vi "AcquireSampleImages.vi"(6 "SampleName":string, 7 "TLCamera reference in":refnum<k24>, 8 "Error In":errorcluster, 9 "Exposure":u16, 10 "Schedule File":path, 11 "MotorController in":refnum<class "MotorController.lvclass">) -> (0 "Error Out":errorcluster, 3 "MotorController out":refnum<class "MotorController.lvclass">, 5 "TLCamera reference out":refnum<k24>)   [LabVIEW 2019]
uses:
  MotorController.lvclass
  C:/Users/jleeman/git_repos/CAxis_Machine/C-Axis LabView Controller/Library_X64/Thorlabs.TSI.TLCameraInterfaces.dll
  Library_X64/Thorlabs.TSI.TLCameraInterfaces.dll
  AcquireSampleImages_states_enum_typedef.ctl
  <vilib>/Utility/file.llb/Read Delimited Spreadsheet (I64).vi
panel:
  in  "Next":bool
  out "Progress":u8(slide) scale=0.0..100.0
  out "Image":u16[][](graph)
  out "Acquisition Schedule":i64[][](array[numeric])
  # "Measure Sample"
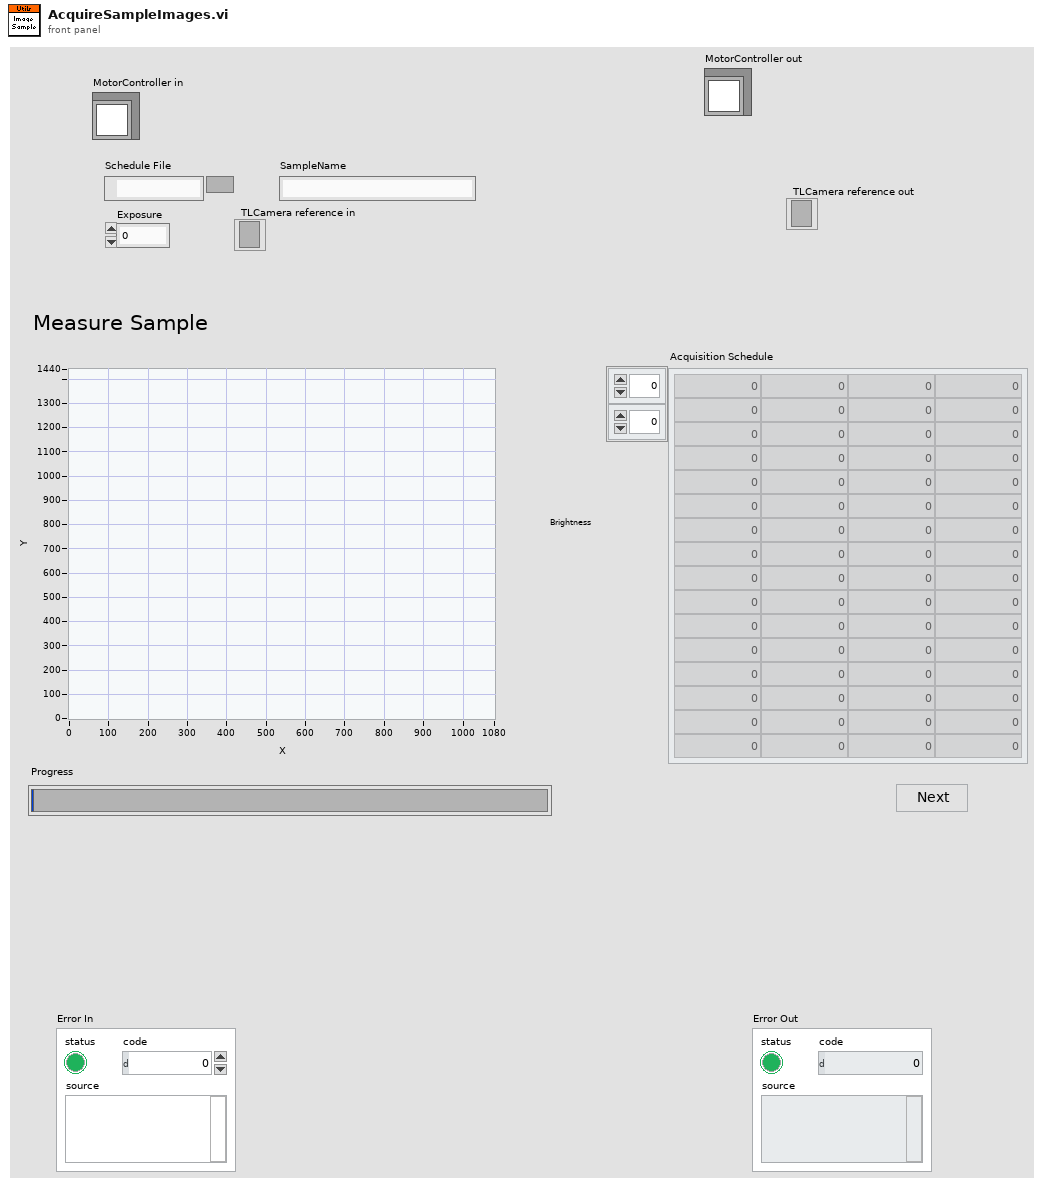
[diagram p1: front panel]
types:
  T1 = enum8{"Enabled", "Disabled", "Disabled and Grayed Out"}
  T2 = typedef "AcquireSampleImages_states_enum_typedef.ctl" = enum16{"Shutdown", "Wait", "TakeImages", "Initialize"}
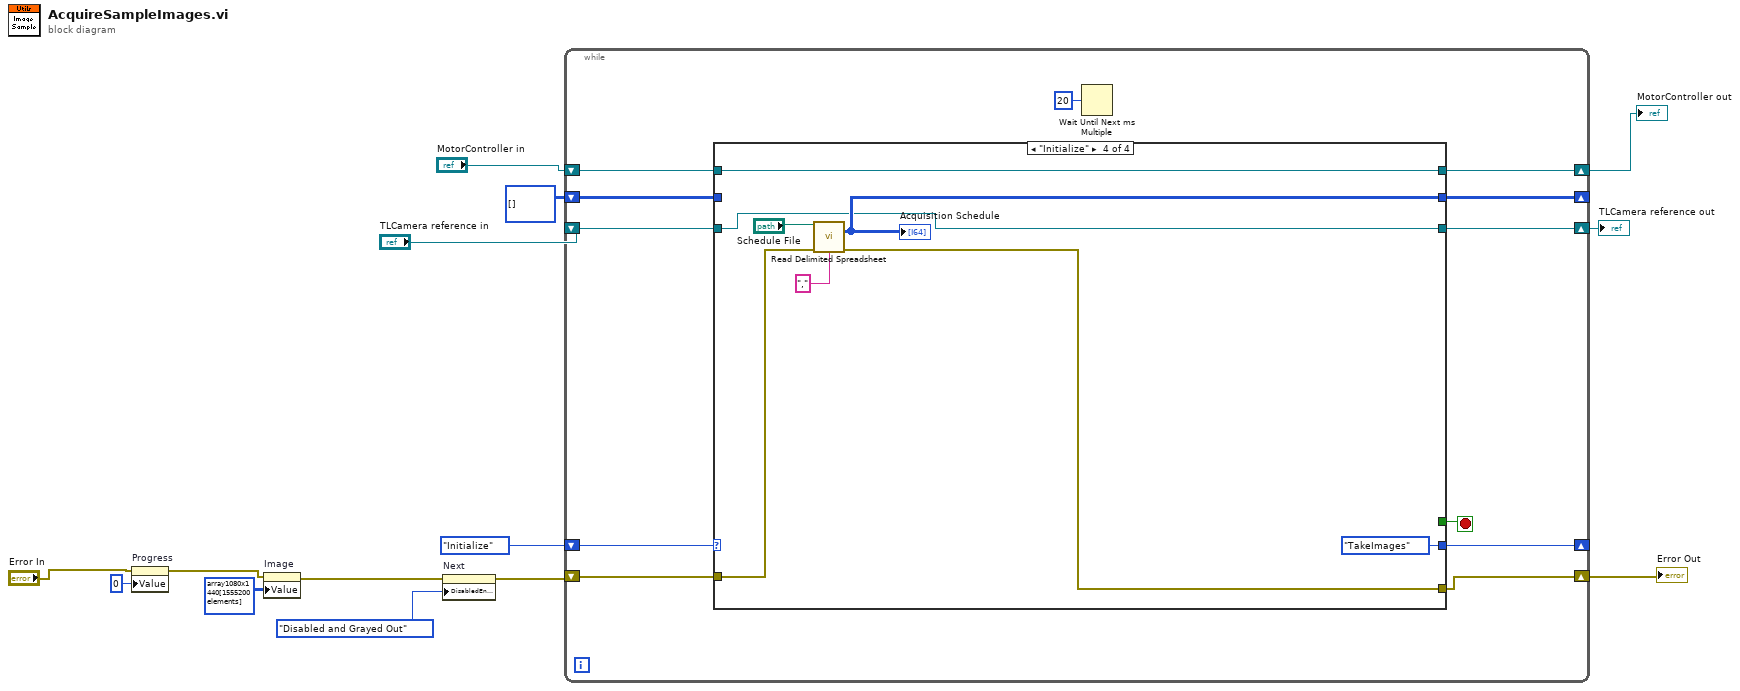
[diagram p0: block diagram]
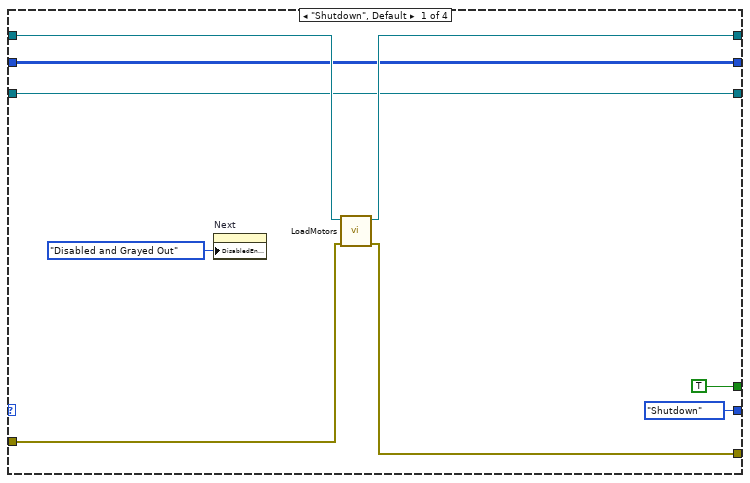
[diagram p2: hidden frame]
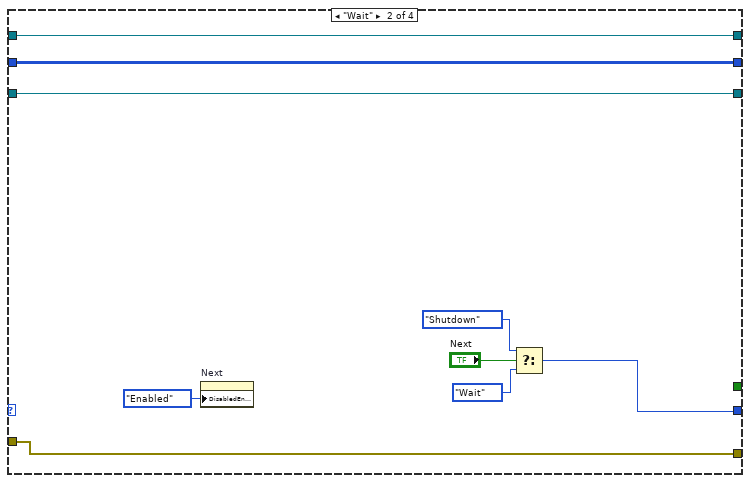
[diagram p3: hidden frame]
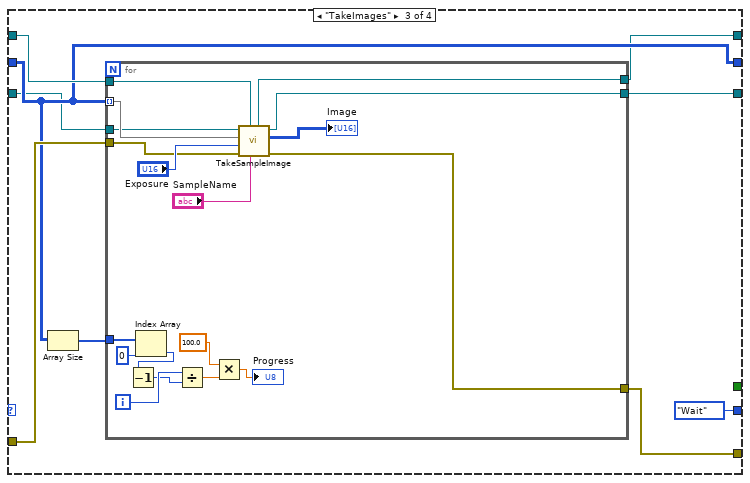
[diagram p4: hidden frame]
diagram:
  n1 = property on="Progress" class="Slide (strict)"(error in="Error In", "Value"=u8 0 ("Progress")) -> (error out=w5:errorcluster)  [unwired: 1 in, 1 out]
  n2 = property on="Image" class="IntGraph (strict)"(error in=w5, "Value"=u16[][] array1080x1440[1555200 elements] ("Image")) -> (error out=w4:errorcluster)  [unwired: 1 in, 1 out]
  n3 = property on="Next" class="Bool"(error in=w4, "DisabledEnum"=T1."Disabled and Grayed Out" ("Disabled")) -> (error out=w12:errorcluster)  [unwired: 1 in, 1 out]
  n4 = while {
    shift-right: [w25] -> _
    shift-left: AcquireSampleImages_states_enum_typedef."Initialize" -> [w26]
    shift-right: [w24] -> _
    shift-left: i64[][] [] ("all rows") -> [w21]
    shift-right: [w22] -> w8
    shift-left: w12 -> [w23]
    shift-right: [w20] -> w10
    shift-left: "MotorController in" -> [w19]
    shift-right: [w18] -> w1
    shift-left: "TLCamera reference in" -> [w17]
    stop <- w15 stop-if-true
    n5 = case shown="\"Initialize\"" w26 {
      tunnel: [AcquireSampleImages_states_enum_typedef."Shutdown" ("f") w41 AcquireSampleImages_states_enum_typedef."Wait" ("f") AcquireSampleImages_states_enum_typedef."TakeImages" ("f")] -> w25
      tunnel: [w31 w40 w49 w76] -> w24
      tunnel: w23 -> [w33 w36 w50 w77]
      tunnel: [w28 w36 w47 w73] -> w22
      tunnel: w21 -> [w31 w40 w49 _]
      tunnel: [w35 w38 w48 w75] -> w20
      tunnel: w19 -> [w34 w38 w51 w75]
      tunnel: [w29 w39 w45 w72] -> w18
      tunnel: w17 -> [w29 w39 w46 w72]
      tunnel: [TRUE _ _ _] -> w15
      frame "Shutdown", Default {
        n6 = property on="Next" class="Bool"("DisabledEnum"=T1."Disabled and Grayed Out" ("Disabled")) -> ()  [unwired: 2 in, 2 out]
        n7 = call "LoadMotors.vi"("error in (no error)"=w33, "MotorController in"=w34) -> ("error out"=w28:errorcluster, "MotorController out"=w35:refnum<class "MotorController.lvclass">)  [unwired: 8 in]
      }
      frame "Wait" {
        n8 = property on="Next" class="Bool"("DisabledEnum"=T1."Enabled" ("Disabled")) -> ()  [unwired: 2 in, 2 out]
        n9 = Select(t=AcquireSampleImages_states_enum_typedef."Shutdown", s="Next", f=AcquireSampleImages_states_enum_typedef."Wait") -> (s? t:f=w41:T2)
      }
      frame "TakeImages" {
        n10 = Array Size(array=w49) -> (size(s)=w53:i32[])
        n11 = for {
          tunnel: w49 -> [w65] mode=indexing
          tunnel: w53 -> [w71]
          tunnel: w51 -> [w67]
          tunnel: w50 -> [w63]
          tunnel: [w66] -> w48
          tunnel: [w62] -> w47
          tunnel: w46 -> [w61]
          tunnel: [w60] -> w45
          i -> [w57]
          n12 = Index Array(array=w71, index=0) -> (element=w55:i32)
          n13 = Decrement(x=w55) -> (x-1=w54:i32)
          n14 = Divide(x=w57, y=w54) -> (x/y=w70:dbl)
          n15 = Multiply(x=100.0, y=w70) -> (x*y=→"Progress":dbl)
          n16 = call "TakeSampleImage.vi"("SampleName"="SampleName", "MotorController in"=w67, "Error In"=w63, "Exposure"="Exposure", "Angles"=w65, "TLCamera reference in"=w61) -> ("Error Out"=w62:errorcluster, "Image Array"=→"Image":u16[][], "TLCamera reference out"=w60:refnum<k24>, "MotorController out"=w66:refnum<class "MotorController.lvclass">)  [unwired: 2 in]
        }
      }
      frame "Initialize" {
        n17 = call-poly <vilib>:"Read Delimited Spreadsheet.vi"("file path (dialog if empty)"="Schedule File", "error in (no error)"=w77, "delimiter (\\t)"="," ("delimiter (\\t)")) -> ("all rows"=w76:i64[][], "error out"=w73:errorcluster)  [unwired: 7 in, 4 out]
        "Acquisition Schedule" <- w76
      }
    }
    n18 = Wait Until Next ms Multiple(millisecond multiple=u32 20) -> ()  [unwired: 1 out]
  }
  "Error Out" <- w8
  "MotorController out" <- w10
  "TLCamera reference out" <- w1
